vi "GetProcessModeParamsNew.vi"(8 "error in (no error)":errorcluster, 10 "Mode":string, 11 "TopLevel in":refnum<class "TopLevel.lvclass">) -> (0 "error out":errorcluster, 2 "ProcessModeValues":T1, 3 "TopLevel out":refnum<class "TopLevel.lvclass">)   [LabVIEW 2022 SP3, in "TopLevel.lvclass"]
uses:
  TopLevel.lvclass
  Typedefs/ProcessModeParamsNew--Cluster.ctl
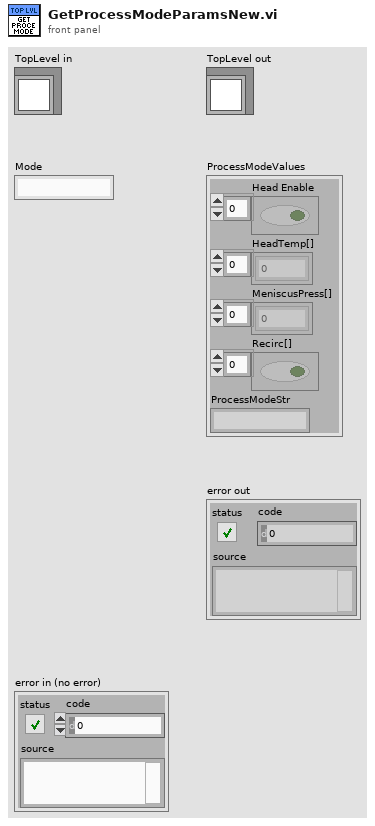
[diagram p1: front panel]
types:
  T1 = typedef "ProcessModeParamsNew--Cluster.ctl" = cluster{"Head Enable":bool[], "HeadTemp[]":dbl[], "MeniscusPress[]":dbl[], "Recirc[]":bool[], "ProcessModeStr":string}
  T2 = cluster{"Name":string, "Heat":dbl, "Meniscus":dbl, "Recirculation":bool}[]
  T3 = typedef "TD Dynamic CVT DVR--ref.ctl" = refnum<data-value>
  T4 = typedef "DLPConfig_Initialization.ctl" = cluster{"PrinterInitialization":cluster{"Printer":cluster{"#attributes":cluster{"Name":string}}, "VacPumpSet":cluster{"#attributes":cluster{"VacPumpEnable":bool, "VacPumpSpeed":dbl}}, "HIBEnable":cluster{"#attributes":cluster{"HIB1Enable":bool, "HIB2Enable":bool, "HIB3Enable":bool, "HIB4Enable":bool, "HIB5Enable":bool, "HIB6Enable":bool}}, "PrinterCompensation":T5}, "HeadSet":cluster{"HeadProperties":T6[]}, "InkSet":cluster{"Ink":T8[]}, "Troubleshooting":cluster{"PMBLogging":cluster{"#attributes":cluster{"PMBMonitorDuringPrint":bool, "PMBMonitorDuringIdle":bool, "LogSwatheInputData":bool, "LogSwatheOutputData":bool, "LogPrintheadColourPlanes":bool, "LogPMBCommunication":bool, "LogSimulatedOutput":bool, "LogAllPMBCommunicationData":bool, "LogPMBSpace":bool, "ExtendedPMBSpaceLogging":bool, "LogPMBWriteSpeed":bool, "LogUsbRetries":bool}}, "HIBLogging":cluster{"#attributes":cluster{"HIBMonitoringDuringPrint":bool, "HIBMonitoringLog":bool}}}}
  T5 = typedef "DLP2_PrinterCompensationProperties.ctl" = cluster{"#attributes":cluster{"AppName":string, "PrintWeightMultiplier":dbl, "Rotation":bool, "Driver":string, "Server":string, "Database":string, "User":string, "Password":string}}
  T6 = typedef "DLP2_PrinterHeadProperties.ctl" = cluster{"#attributes":T7}
  T7 = typedef "DLPConfig)Init_HeadPropertyAttr--Cluster.ctl" = cluster{"HeadNumber":u8, "Material":string, "HeadLocalX":dbl, "HeadLocalY":dbl, "HeadRotationAngle":dbl, "VH2L_Hi":dbl, "VH2R_Hi":dbl, "VH1LA_Hi":dbl, "VH1LB_Hi":dbl, "VH1RA_Hi":dbl, "VH1RB_Hi":dbl, "VH2L_Lo":dbl, "VH2R_Lo":dbl, "VH1LA_Lo":dbl, "VH1LB_Lo":dbl, "VH1RA_Lo":dbl, "VH1RB_Lo":dbl}
  T8 = typedef "DLP2_PrinterMaterialProperties.ctl" = cluster{"#attributes":cluster{"InkType":string, "PrePrintPurge":bool, "PurgeTime":dbl, "PurgeCount":i32, "Density":dbl, "NumberofDrops":i32, "PrintWeight":dbl, "PrintheadPrime":bool}, "Idle":cluster{"Name":string, "Heat":dbl, "Meniscus":dbl, "Recirculation":bool}[], "Process":cluster{"Name":string, "Heat":dbl, "Meniscus":dbl, "Recirculation":bool, "ColorPlane":string}[]}
  T9 = cluster{"HIB1Enable":bool, "HIB2Enable":bool, "HIB3Enable":bool, "HIB4Enable":bool, "HIB5Enable":bool, "HIB6Enable":bool}
  T10 = cluster{"Name":string, "Heat":dbl, "Meniscus":dbl, "Recirculation":bool, "ColorPlane":string}[]
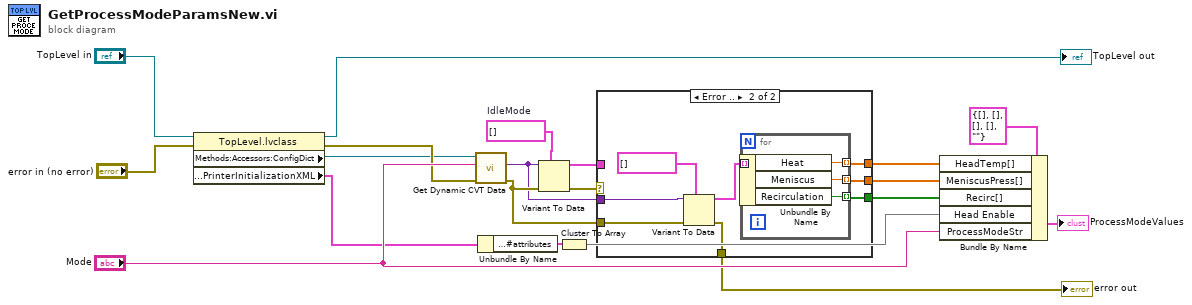
[diagram p0: block diagram]
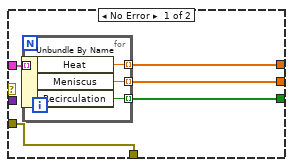
[diagram p2: hidden frame]
diagram:
  w3 = T2 []  # IdleMode
  n1 = property class="TopLevel.lvclass"(reference="TopLevel in", error in="error in (no error)") -> (reference out=→"TopLevel out":refnum<class "TopLevel.lvclass">, error out=w12:errorcluster, "Methods:Accessors:ConfigDict"=w2:T3, "Methods:Accessors:PrinterInitializationXML"=w8:T4)
  n2 = call <vilib>:"Get Dynamic CVT Data.vi"("error in (no error)"=w12, "DataName"="Mode", "dCVT DVR"=w2) -> ("error out"=w6:errorcluster, "value"=w5:variant)  [unwired: 5 in, 2 out]
  n3 = Unbundle By Name(w8) -> ("PrinterInitialization.HIBEnable.#attributes"=w9:T9)
  n4 = Variant To Data(error in=w6, type=w3, Variant=w5) -> (data=w7:T2, error out=w4:errorcluster)
  n5 = Cluster To Array(cluster=w9) -> (array=w20:bool[])
  n6 = case shown="Error .." w4 {
    tunnel: w5 -> [_ w36]
    tunnel: w6 -> [w21 w35]
    tunnel: w7 -> [w25 _]
    tunnel: [w24 w33] -> w17
    tunnel: [w23 w32] -> w18
    tunnel: [w22 w31] -> w19
    tunnel: [w21 w30] -> w10
    frame No Error {
      n7 = for {
        tunnel: w25 -> [w29] mode=indexing
        tunnel: [w28] -> w24 mode=indexing
        tunnel: [w27] -> w23 mode=indexing
        tunnel: [w26] -> w22 mode=indexing
        n8 = Unbundle By Name(w29) -> ("Heat"=w28:dbl, "Meniscus"=w27:dbl, "Recirculation"=w26:bool)
      }
    }
    frame Error {
      n9 = Variant To Data(error in=w35, type=T10 [], Variant=w36) -> (data=w34:T10, error out=w30:errorcluster)
      n10 = for {
        tunnel: w34 -> [w41] mode=indexing
        tunnel: [w40] -> w33 mode=indexing
        tunnel: [w39] -> w32 mode=indexing
        tunnel: [w38] -> w31 mode=indexing
        n11 = Unbundle By Name(w41) -> ("Heat"=w40:dbl, "Meniscus"=w39:dbl, "Recirculation"=w38:bool)
      }
    }
  }
  "error out" <- w10
  n12 = Bundle By Name(cluster=T1 {"Head Enable"=[], "HeadTemp[]"=[], "MeniscusPress[]"=[], "Recirc[]"=[], "ProcessModeStr"=""} ("ProcessModeValues"), "HeadTemp[]"=w17, "MeniscusPress[]"=w18, "Recirc[]"=w19, "Head Enable"=w20, "ProcessModeStr"="Mode") -> (→"ProcessModeValues":T1)
